vi "WD_SWA_add_new.vi"(8 "error in (no error)":errorcluster, 10 "New data":cluster{"條碼A":string, "條碼B":string}, 11 "DBLink":string="Driver={ODBC Driver 17 for SQL Server};Server=localhost\\SQLEXPRESS;Database=ZDX201;UID=labview;PWD=Dsa@54137926") -> (0 "error out":errorcluster, 1 "站點總數":i32, 2 "當前料數":i32, 3 "計算用 array":cluster{"條碼A":string, "條碼B":string}[](array[cluster]), 5 "顯示用array":cluster{"條碼A":string, "條碼B":string}[](array[cluster]))   [LabVIEW 2019]
panel:
  out "x-y":i32
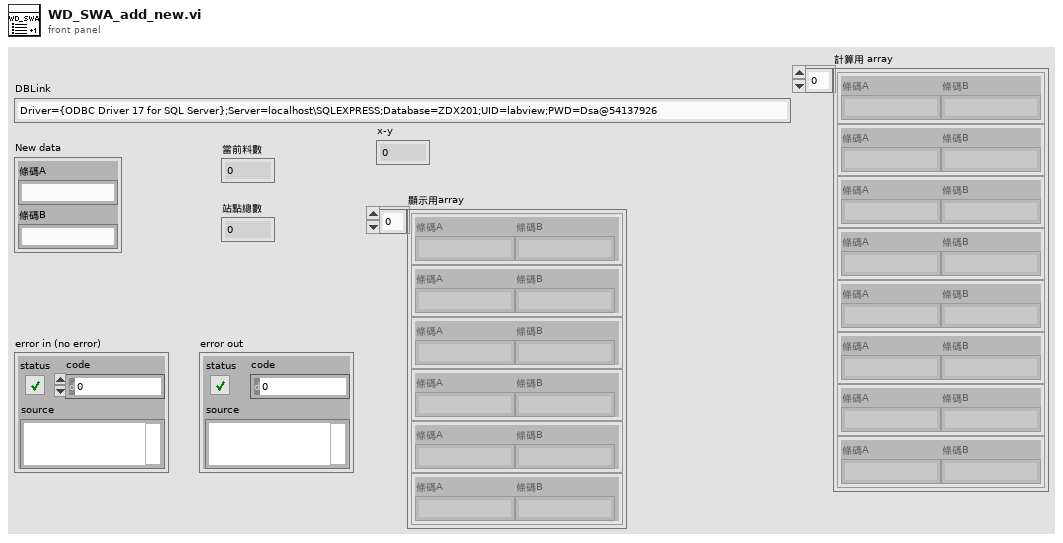
[diagram p1: front panel]
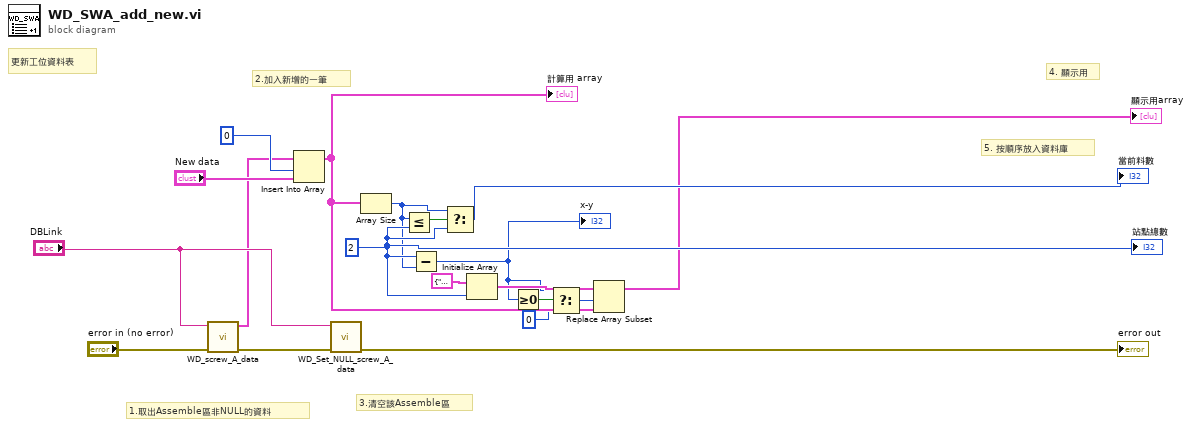
[diagram p0: block diagram]
diagram:
  w13 = 2
  # "5. 按順序放入資料庫"
  # "4. 顯示用"
  # "3.清空該Assemble區"
  # "2.加入新增的一筆"
  # "1.取出Assemble區非NULL的資料"
  # "更新工位資料表"
  n1 = call "WD_screw_A_data.vi"("error in (no error)"="error in (no error)", "DBlink"="DBLink") -> ("error out"=w3:errorcluster, "鎖A備料"=w1:cluster{"條碼A":string, "條碼B":string}[])  [unwired: 6 in, 2 out]
  n2 = Insert Into Array(array=w1, index=0, new element="New data") -> (w14:cluster{"條碼A":string, "條碼B":string}[])
  "計算用 array" <- w14
  n3 = call "WD_Set_NULL_screw_A_data.vi"("error in (no error)"=w3, "DBlink"="DBLink") -> ("error out"=→"error out":errorcluster)  [unwired: 8 in, 1 out]
  n4 = Array Size(array=w14) -> (size(s)=w12:i32)
  n5 = Less Or Equal?(x=w12, y=w13) -> (x <= y?=w18:bool)
  n6 = Subtract(x=w13, y=w12) -> (x-y=w7:i32)
  "x-y" <- w7
  n7 = Select(t=w12, s=w18, f=w13) -> (s? t:f=→"當前料數":i32)
  n8 = Initialize Array(cluster{"條碼A":string, "條碼B":string} {"條碼A"="NULL", "條碼B"="NULL"} ("New data"), w13) -> (w15:cluster{"條碼A":string, "條碼B":string}[])
  n9 = Greater Or Equal To 0?(x=w7) -> (x >= 0?=w9:bool)
  n10 = Select(t=w7, s=w9, f=i16 0) -> (s? t:f=w6:i32)
  n11 = Replace Array Subset(array=w15, new element=w14, index=w6) -> (→"顯示用array":cluster{"條碼A":string, "條碼B":string}[])
  "站點總數" <- w13
